vi "Set Stop Button Status.vi"(8 "Error In":errorcluster, 11 "Stop Button":bool) -> (0 "Error Out":errorcluster)   [LabVIEW 2019]
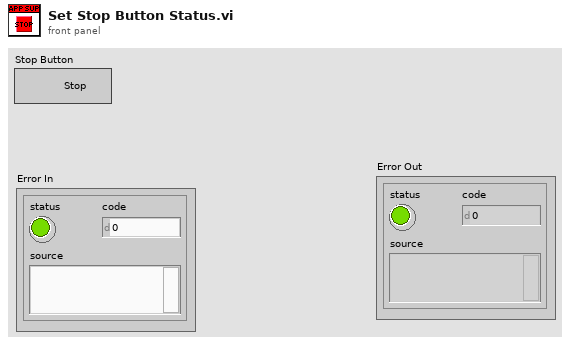
[diagram p1: front panel]
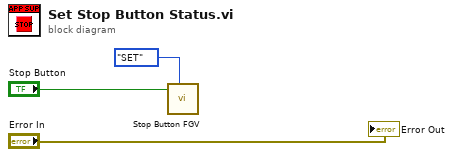
[diagram p0: block diagram]
diagram:
  n1 = call "Stop Button FGV.vi"("Operation"=enum16{"GET", "SET"}."SET", "Stop Button"="Stop Button") -> ()  [unwired: 9 in, 1 out]
  "Error Out" <- "Error In"
